vi "GetType.vi"(8 "error in (no error)":errorcluster, 11 "Set Mode Msg":refnum<class "Set Mode Msg.lvclass">) -> (0 "error out":errorcluster, 2 "Data Sample":variant, 3 "Set Mode Msg":refnum<class "Set Mode Msg.lvclass">)   [LabVIEW 2016, in "CS++PPG.lvlib" / "Set Mode Msg.lvclass"]
uses:
  Set Mode Msg.lvclass
  Set Mode Msg.lvclass/Set Mode Msg.ctl
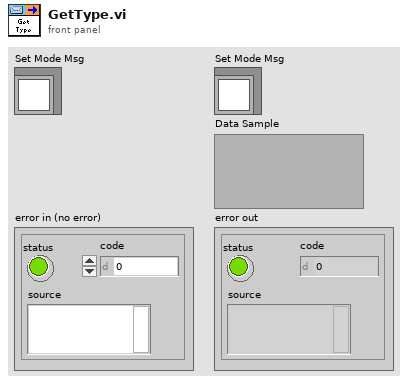
[diagram p1: front panel]
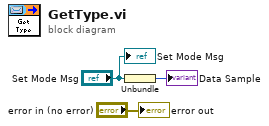
[diagram p0: block diagram]
diagram:
  n1 = Unbundle("Set Mode Msg") -> (→"Data Sample":u8)
  "error out" <- "error in (no error)"
  "Set Mode Msg" <- "Set Mode Msg"
